vi "niusrprios Configure Tx.vi"(0 "niUsrpRio Session":T1={"FPGA Interface"=refnum, "RIO Interface Number"=0, "Data Clock Rate"=0, "FPGA Data Clock Rate"=0, "Global Settings Register Bus"=refnum, "Radio 0 Settings Register Bus"=refnum, "Radio 1 Settings Register Bus"=refnum, "Radio Settings Bus Semaphore"=refnum, "DB Queues"=[], "Characterization Data Valid?"=FALSE, "EEPROM Header"={"Checksum"=0, "Product Code"=0, "Hardware Current Version"=0, "Hardware Oldest Compatible Version"=0, "EEPROM Map Current Version"=0, "EEPROM Map Oldest Compatible Version"=0, "User Password"="", "Pointer to Factory Header"=0, "Pointer to User Header"=0, "Recommended Interval"=0, "Number of Reserved Bytes"=9, "Number of Daughterboards"=0, "Daughterboard IDs"=[], "Daughterboard Serial Numbers"=[]}, "Device Data Header"={"Checksum"=0, "Number of Channels"=0, "Number of Gain Settings"=[], "Pointer to Characterization Data"=[], "Number of Reserved Bytes"=27, "Number of Frequencies"=[]}, "EEPROM Characterization Header"={"Checksum"=0, "Date"=timestamp(0 s since 1904-01-01), "Temperature"=0.0, "Misc. Info"="", "Pointer to Device Data Header"=0, "Number of Reserved Bytes"=28}, "Characterization Data"=[], "FPGA Current Version"=0, "FPGA Oldest Compatible Version"=0, "Fixed Logic Current Version"=0, "Fixed Logic Oldest Compatible Version"=0, "FPGA Radio Settings Bus Current Version"=0, "FPGA Radio Settings Bus Oldest Compatible Version"=0, "FPGA Board Config Current Version"=0, "FPGA Board Config Oldest Compatible Version"=0, "Daughterboard Clock Rate"=0} {"Daughterboard Clock Rate" format="%#.3pHz"; "FPGA Data Clock Rate" format="%#.3pHz"; "Data Clock Rate" format="%#.3pHz"; "Characterization Data"."Frequencies [Hz]" format="%#_6p"; "EEPROM Characterization Header"."Pointer to Device Data Header" format="%x"; "EEPROM Characterization Header"."Checksum" format="%x"; "Device Data Header"."Pointer to Characterization Data" format="%x"; "Device Data Header"."Checksum" format="%x"; "EEPROM Header"."Pointer to User Header" format="%x"; "EEPROM Header"."Pointer to Factory Header" format="%x"; "EEPROM Header"."Product Code" format="%x"; "EEPROM Header"."Checksum" format="%x"}, 5 "tx config":T11={"rf enable 0"=FALSE, "rf config 0"={"antenna"="TX1", "frequency"=2000000000.0, "lo frequency"=-1.0, "level"=0.0}, "rf enable 1"=FALSE, "rf config 1"={"antenna"="TX1", "frequency"=2000000000.0, "lo frequency"=-1.0, "level"=0.0}, "transfer mode"=enum."Finite", "sample rate"=10000000.0, "number of samples"=8192, "start trigger"=enum."Immediate", "tone frequency"=100000.0} {"tone frequency" format="%#.3pHz"; "sample rate" format="%#.3pS/s"; "rf config 0"."level" format="%#_gdBm"; "rf config 0"."lo frequency" format="%#.3pHz"; "rf config 0"."frequency" format="%#.3pHz"; "rf config 1"."level" format="%#_gdBm"; "rf config 1"."lo frequency" format="%#.3pHz"; "rf config 1"."frequency" format="%#.3pHz"}, 11 "error in":errorcluster) -> (4 "niUsrpRio Session (out)":T1 {"Daughterboard Clock Rate" format="%#.3pHz"; "FPGA Data Clock Rate" format="%#.3pHz"; "Data Clock Rate" format="%#.3pHz"; "Characterization Data"."Frequencies [Hz]" format="%#_6p"; "EEPROM Characterization Header"."Pointer to Device Data Header" format="%x"; "EEPROM Characterization Header"."Checksum" format="%x"; "Device Data Header"."Pointer to Characterization Data" format="%x"; "Device Data Header"."Checksum" format="%x"; "EEPROM Header"."Pointer to User Header" format="%x"; "EEPROM Header"."Pointer to Factory Header" format="%x"; "EEPROM Header"."Product Code" format="%x"; "EEPROM Header"."Checksum" format="%x"}, 6 "tx.enabled channels":string[](array[string]), 8 "I":i16[](array[numeric]), 10 "Q":i16[](array[numeric]), 13 "tx.output waveform":waveform(dbl)[](graph), 14 "tx.coerced configurations":T12 {"coerced sample rates" format="%#.3pS/s"; "coerced levels" format="%#.3gdBm"; "coerced lo frequencies" format="%#.3pHz"; "coerced frequencies" format="%#.3pHz"}, 15 "error out":errorcluster)   [LabVIEW 2015]
uses:
  <instrlib>/niUsrpRio/Config/v1/Host/Public/niUsrpRio Session.ctl
  <instrlib>/_niInstr/Register Bus/v0/Host/Public/Register Bus Session.ctl
  <instrlib>/_niInstr/Register Bus/v0/Host/Private/Session Data.ctl
  <instrlib>/niUsrpRio/Config/v1/Host/Private/DB Queue Reference.ctl
  <instrlib>/niUsrpRio/Config/v1/Host/Private/Daughterboard Data.ctl
  <instrlib>/niUsrpRio/Config/v1/Host/Private/ATR state data.ctl
  <instrlib>/niUsrpRio/Config/v1/Host/Private/Antenna Configuration.ctl
  <instrlib>/niUsrpRio/Config/v1/Host/Private/CPLD Power Mode.ctl
  <instrlib>/niUsrpRio/Config/v1/Host/Public/EEPROM Header.ctl
  <instrlib>/niUsrpRio/Config/v1/Host/Public/EEPROM Device Data Header.ctl
  <instrlib>/niUsrpRio/Config/v1/Host/Public/EEPROM Characterization Header.ctl
  <instrlib>/niUsrpRio/Config/v1/Host/Public/Characterization Data.ctl
  <instrlib>/niUsrpRio/Config/v1/Host/Public/IQ Imbalance.ctl
  niusrprios Start Trigger.ctl
  niusrprios Configure Signal (Level).vi
  <instrlib>/_niInstr/Register Bus/v0/Host/niInstr Register Bus v0 Host.lvlib
  <instrlib>/niUsrpRio/Config/v1/Host/niUsrpRio Config v1 Host.lvlib
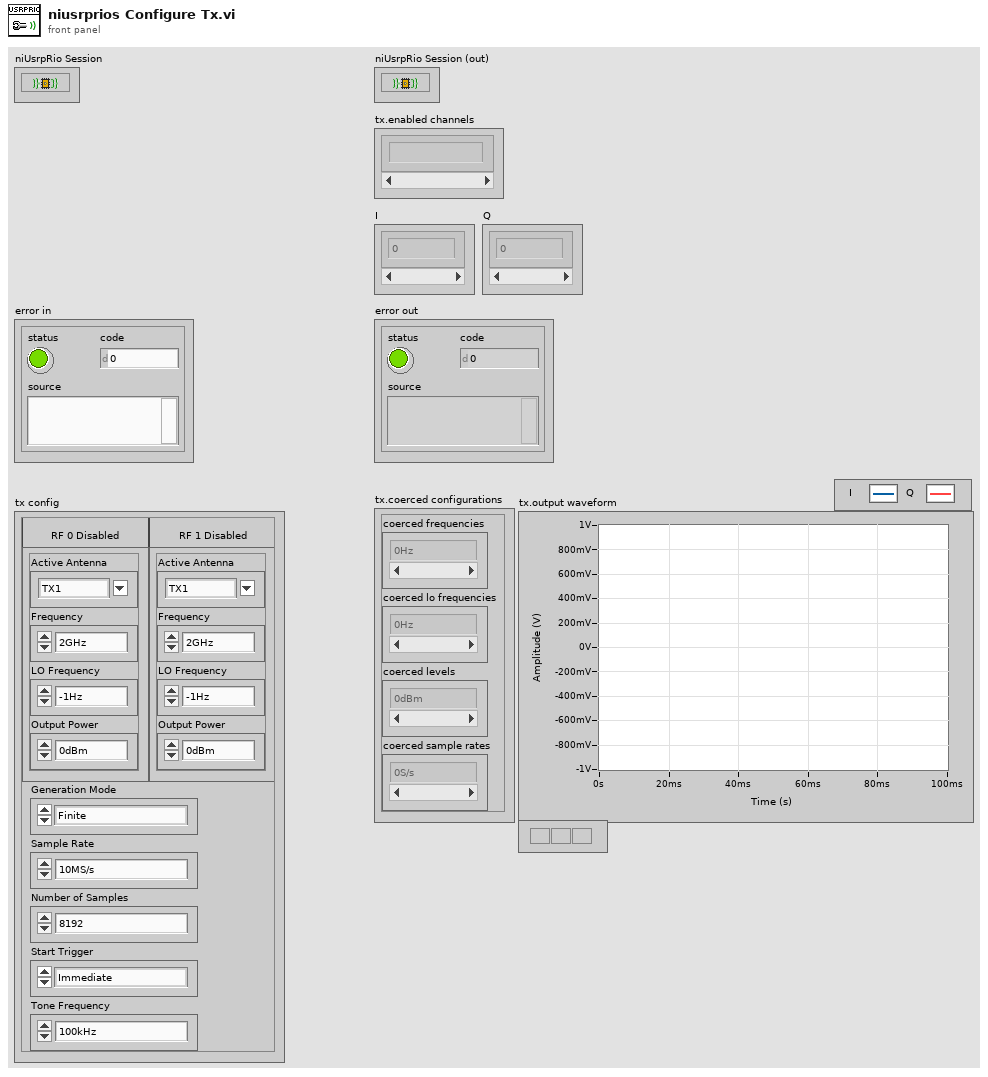
[diagram p1: front panel]
types:
  T1 = typedef "niUsrpRio Config v1 Host.lvlib/niUsrpRio Session.ctl" = cluster{"FPGA Interface":refnum<k20>, "RIO Interface Number":u32, "Data Clock Rate":u32, "FPGA Data Clock Rate":u32, "Global Settings Register Bus":T2, "Radio 0 Settings Register Bus":T2, "Radio 1 Settings Register Bus":T2, "Radio Settings Bus Semaphore":T3, "DB Queues":T4[], "Characterization Data Valid?":bool, "EEPROM Header":T5, "Device Data Header":T6, "EEPROM Characterization Header":T7, "Characterization Data":T8[], "FPGA Current Version":u32, "FPGA Oldest Compatible Version":u32, "Fixed Logic Current Version":u32, "Fixed Logic Oldest Compatible Version":u32, "FPGA Radio Settings Bus Current Version":u32, "FPGA Radio Settings Bus Oldest Compatible Version":u32, "FPGA Board Config Current Version":u32, "FPGA Board Config Oldest Compatible Version":u32, "Daughterboard Clock Rate":u32}
  T2 = typedef "niInstr Register Bus v0 Host.lvlib/Register Bus Session.ctl" = refnum<queue>
  T3 = typedef "Semaphore RefNum" = refnum<k1>
  T4 = typedef "niUsrpRio Config v1 Host.lvlib/DB Queue Reference.ctl" = refnum<queue>
  T5 = typedef "niUsrpRio Config v1 Host.lvlib/EEPROM Header.ctl" = cluster{"Checksum":u32, "Product Code":u16, "Hardware Current Version":u16, "Hardware Oldest Compatible Version":u16, "EEPROM Map Current Version":u16, "EEPROM Map Oldest Compatible Version":u16, "User Password":string, "Pointer to Factory Header":u32, "Pointer to User Header":u32, "Recommended Interval":u16, "Number of Reserved Bytes":i32, "Number of Daughterboards":u8, "Daughterboard IDs":u16[], "Daughterboard Serial Numbers":string[]}
  T6 = typedef "niUsrpRio Config v1 Host.lvlib/EEPROM Device Data Header.ctl" = cluster{"Checksum":u32, "Number of Channels":u8, "Number of Gain Settings":u16[], "Pointer to Characterization Data":u32[], "Number of Reserved Bytes":i32, "Number of Frequencies":u16[]}
  T7 = typedef "niUsrpRio Config v1 Host.lvlib/EEPROM Characterization Header.ctl" = cluster{"Checksum":u32, "Date":timestamp, "Temperature":sgl, "Misc. Info":string, "Pointer to Device Data Header":u32, "Number of Reserved Bytes":i32}
  T8 = typedef "niUsrpRio Config v1 Host.lvlib/Characterization Data.ctl" = cluster{"Gains[dB]":dbl[], "Frequencies [Hz]":dbl[], "IQ Imbalance Table":T9[], "Measured Gains[dB]":dbl[][]}
  T9 = typedef "niUsrpRio Config v1 Host.lvlib/IQ Imbalance.ctl" = cluster{"Gain Imbalance [linear]":dbl, "Phase Imbalance [radians]":dbl, "Offset":cdb}
  T10 = typedef "niusrprios Start Trigger.ctl" = enum8{"Software", "Digital Edge", "Rx Start Trigger", "Tx Start Trigger", "Immediate", "Future Time Event"}
  T11 = cluster{"rf enable 0":bool, "rf config 0":cluster{"antenna":string, "frequency":dbl, "lo frequency":dbl, "level":dbl}, "rf enable 1":bool, "rf config 1":cluster{"antenna":string, "frequency":dbl, "lo frequency":dbl, "level":dbl}, "transfer mode":enum16{"Finite", "Continuous"}, "sample rate":dbl, "number of samples":u32, "start trigger":T10, "tone frequency":dbl}
  T12 = cluster{"coerced frequencies":dbl[], "coerced lo frequencies":dbl[], "coerced levels":dbl[], "coerced sample rates":dbl[]}
  T13 = cluster{"antenna":string, "frequency":dbl, "lo frequency":dbl, "level":dbl}
  T14 = cluster{"rf enable 0":bool, "rf config 0":cluster{"antenna":string, "frequency":dbl, "lo frequency":dbl, "level":dbl}}
  T15 = cluster{"rf enable 1":bool, "rf config 1":cluster{"antenna":string, "frequency":dbl, "lo frequency":dbl, "level":dbl}}
  T16 = cluster{"rf enable 1":bool, "rf config 1":cluster{"antenna":string, "frequency":dbl, "lo frequency":dbl, "level":dbl}}[]
  T17 = cluster{"antenna":string, "frequency":dbl, "lo frequency":dbl, "level":dbl}[]
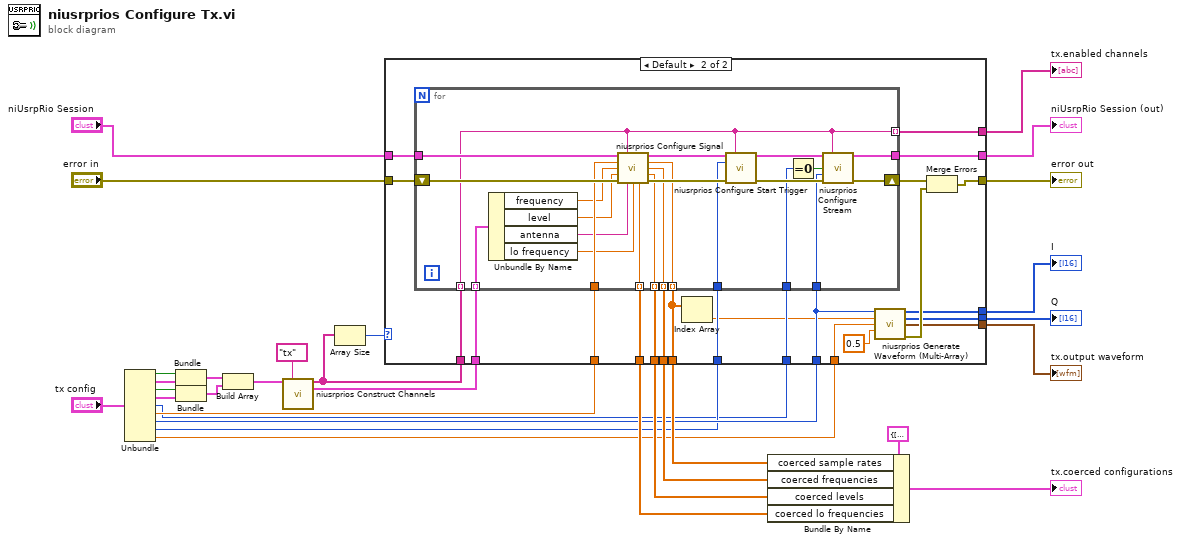
[diagram p0: block diagram]
diagram:
  n1 = Unbundle("tx config") -> ("rf enable 0"=w18:bool, "rf config 0"=w17:T13, "rf enable 1"=w16:bool, "rf config 1"=w15:T13, "transfer mode"=w6:enum16{"Finite", "Continuous"}, "sample rate"=w14:dbl, "number of samples"=w8:u32, "start trigger"=w7:T10, "tone frequency"=w5:dbl)
  n2 = Bundle("rf enable 0"=w18, "rf config 0"=w17) -> (w26:T14)  [unwired: 1 in]
  n3 = Bundle("rf enable 1"=w16, "rf config 1"=w15) -> (w25:T15)  [unwired: 1 in]
  n4 = Build Array(w26, w25) -> (w23:T16)
  n5 = call "niusrprios Construct Channels.vi"("channel configurations"=w23, "scope"="tx") -> ("enabled channels"=w9:string[], "enabled channel configurations"=w24:T17)  [unwired: 12 in]
  n6 = Array Size(array=w9) -> (size(s)=w10:i32)
  n7 = case shown="Default" w10 {
    tunnel: [_ w35] -> w31
    tunnel: [_ w56] -> w30
    tunnel: [_ w55] -> w29
    tunnel: [_ w54] -> w28
    tunnel: w7 -> [_ w53]
    tunnel: w9 -> [_ w52]
    tunnel: w24 -> [_ w51]
    tunnel: [_ w50] -> w22
    tunnel: w14 -> [_ w43]
    tunnel: w6 -> [_ w49]
    tunnel: w8 -> [_ w42]
    tunnel: [w33 w48] -> w13
    tunnel: "error in" -> [w32 w47]
    tunnel: "niUsrpRio Session" -> [w33 w46]
    tunnel: [w32 w40] -> w27
    tunnel: w5 -> [_ w44]
    tunnel: [_ w38] -> w4
    tunnel: [_ w37] -> w3
    tunnel: [_ w36] -> w2
    frame 0 {
    }
    frame Default {
      n8 = for "channel configuration" {
        tunnel: [w73] -> w54 mode=indexing
        tunnel: w53 -> [w75]
        tunnel: w42 -> [w59]
        tunnel: w49 -> [w74]
        shift-right: [w58] -> w45
        shift-left: w47 -> [w79]
        tunnel: w43 -> [w78]
        tunnel: [w72] -> w55 mode=indexing
        tunnel: [w71] -> w56 mode=indexing
        tunnel: [w70] -> w35 mode=indexing
        tunnel: w51 -> [w69] mode=indexing
        tunnel: w52 -> [w66] mode=indexing
        tunnel: [w66] -> w50 mode=indexing
        tunnel: [w68] -> w48
        tunnel: w46 -> [w67]
        n9 = Unbundle By Name(w69) -> ("frequency"=w63:dbl, "level"=w60:dbl, "antenna"=w62:string, "lo frequency"=w61:dbl)
        n10 = call-poly "niusrprios Configure Signal.vi"("niUsrpRio Session"=w67, "scope"=w66, "sample rate [S/s]"=w78, "frequency [Hz]"=w63, "level [dBm]"=w60, "error in"=w79, "Active Antenna"=w62, "LO frequency [Hz]"=w61) -> ("niUsrpRio Session (out)"=w65:T1, "coerced sample rate [S/s]"=w70:dbl, "coerced frequency [Hz]"=w71:dbl, "coerced level [dBm]"=w72:dbl, "coerced LO frequency [Hz]"=w73:dbl, "error out"=w77:errorcluster)  [unwired: 1 in, 1 out]
        n11 = call "niusrprios Configure Start Trigger.vi"("niUsrpRio Session"=w65, "scope"=w66, "start trigger"=w75, "error in"=w77) -> ("niUsrpRio Session (out)"=w64:T1, "error out"=w76:errorcluster)  [unwired: 10 in]
        n12 = Equal To 0?(x=w74) -> (x = 0?=w57:bool)
        n13 = call "niusrprios Configure Stream.vi"("niUsrpRio Session"=w64, "scope"=w66, "number of samples is finite"=w57, "number of samples"=w59, "error in"=w76) -> ("niUsrpRio Session (out)"=w68:T1, "error out"=w58:errorcluster)  [unwired: 9 in]
      }
      n14 = Index Array(array=w35) -> (element=w34:dbl)  [unwired: 1 in]
      n15 = call "niusrprios Generate Waveform (Multi-Array).vi"("number of samples"=w42, "sample rate"=w34, "tone frequency"=w44, "amplitude"=0.5) -> ("I"=w38:i16[], "Q"=w37:i16[], "Waveform"=w36:waveform(dbl)[], "error out"=w39:errorcluster)  [unwired: 8 in]
      n16 = Merge Errors(w45, w39) -> (w40:errorcluster)
    }
  }
  "niUsrpRio Session (out)" <- w13
  "error out" <- w27
  "tx.enabled channels" <- w22
  "tx.output waveform" <- w2
  "I" <- w4
  "Q" <- w3
  n17 = Bundle By Name(cluster=T12 {"coerced frequencies"=[], "coerced lo frequencies"=[], "coerced levels"=[], "coerced sample rates"=[]} ("coerced configurations"), "coerced sample rates"=w31, "coerced frequencies"=w30, "coerced levels"=w29, "coerced lo frequencies"=w28) -> (→"tx.coerced configurations":T12)
